vi "controllerVoltage.vi"(8 "error in (no error)":errorcluster) -> (0 "error out":errorcluster)   [LabVIEW 2018]
uses:
  Global_1259.vi
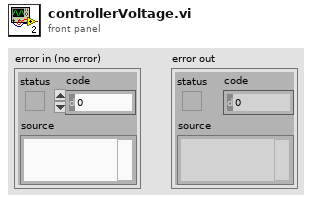
[diagram p1: front panel]
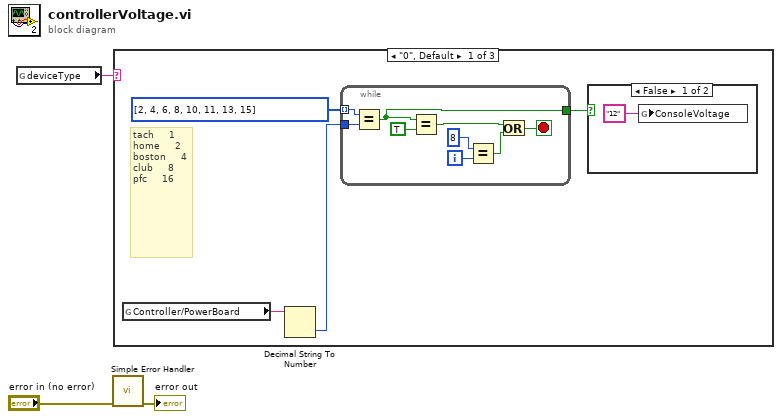
[diagram p0: block diagram]
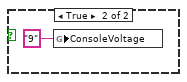
[diagram p2: hidden frame]
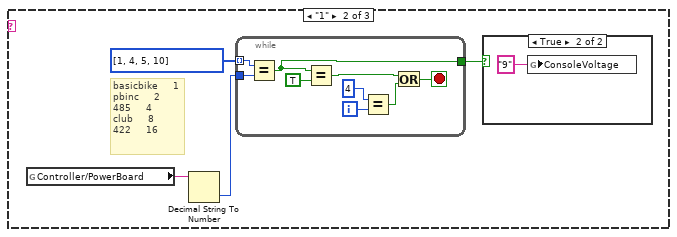
[diagram p3: hidden frame]
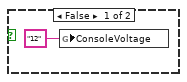
[diagram p4: hidden frame]
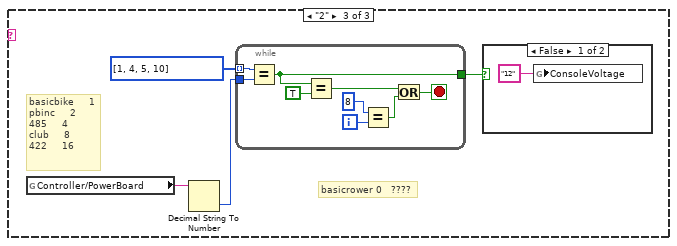
[diagram p5: hidden frame]
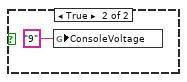
[diagram p6: hidden frame]
diagram:
  n1 = global read "Global_1259.vi" "deviceType"() -> (w3:string)
  n2 = call <vilib>:"Simple Error Handler.vi"("error in (no error)"="error in (no error)") -> ("error out"=→"error out":errorcluster)  [unwired: 4 in, 4 out]
  n3 = case shown="\"0\", Default" w3 {
    frame "0", Default {
      # "tach     1\nhome     2\nboston     4\nclub     8\npfc     16"
      n4 = global read "Global_1259.vi" "Controller/PowerBoard"() -> (w4:string)
      n5 = Decimal String To Number(string=w4) -> (number=w6:i32)  [unwired: 2 in, 1 out]
      n6 = while {
        tunnel: i32[] [2, 4, 6, 8, 10, 11, 13, 15] -> [w18] mode=indexing
        tunnel: w6 -> [w17]
        tunnel: [w10] -> w5
        i -> [w13]
        stop <- w11 stop-if-true
        n7 = Equal?(x=w18, y=w17) -> (x = y?=w10:bool)
        n8 = Equal?(x=w10, y=TRUE) -> (x = y?=w14:bool)
        n9 = Equal?(x=8, y=w13) -> (x = y?=w15:bool)
        n10 = Or(x=w14, y=w15) -> (x .or. y?=w11:bool)
      }
      n11 = case shown="False" w5 {
        frame False {
          n12 = global write "Global_1259.vi" "ConsoleVoltage"("12" ("ConsoleVoltage")) -> ()
        }
        frame True {
          n13 = global write "Global_1259.vi" "ConsoleVoltage"("9" ("ConsoleVoltage")) -> ()
        }
      }
    }
    frame "1" {
      # "basicbike     1\npbinc     2\n485     4\nclub     8\n422     16"
      n14 = global read "Global_1259.vi" "Controller/PowerBoard"() -> (w19:string)
      n15 = Decimal String To Number(string=w19) -> (number=w21:i32)  [unwired: 2 in, 1 out]
      n16 = while {
        tunnel: i32[] [1, 4, 5, 10] -> [w33] mode=indexing
        tunnel: w21 -> [w32]
        tunnel: [w25] -> w20
        i -> [w28]
        stop <- w26 stop-if-true
        n17 = Equal?(x=w33, y=w32) -> (x = y?=w25:bool)
        n18 = Equal?(x=w25, y=TRUE) -> (x = y?=w29:bool)
        n19 = Equal?(x=4, y=w28) -> (x = y?=w30:bool)
        n20 = Or(x=w29, y=w30) -> (x .or. y?=w26:bool)
      }
      n21 = case shown="True" w20 {
        frame False {
          n22 = global write "Global_1259.vi" "ConsoleVoltage"("12" ("ConsoleVoltage")) -> ()
        }
        frame True {
          n23 = global write "Global_1259.vi" "ConsoleVoltage"("9" ("ConsoleVoltage")) -> ()
        }
      }
    }
    frame "2" {
      # "basicrower 0   ????"
      # "basicbike     1\npbinc     2\n485     4\nclub     8\n422     16"
      n24 = global read "Global_1259.vi" "Controller/PowerBoard"() -> (w34:string)
      n25 = Decimal String To Number(string=w34) -> (number=w36:i32)  [unwired: 2 in, 1 out]
      n26 = while {
        tunnel: i32[] [1, 4, 5, 10] -> [w48] mode=indexing
        tunnel: w36 -> [w47]
        tunnel: [w40] -> w35
        i -> [w43]
        stop <- w41 stop-if-true
        n27 = Equal?(x=w48, y=w47) -> (x = y?=w40:bool)
        n28 = Equal?(x=w40, y=TRUE) -> (x = y?=w44:bool)
        n29 = Equal?(x=8, y=w43) -> (x = y?=w45:bool)
        n30 = Or(x=w44, y=w45) -> (x .or. y?=w41:bool)
      }
      n31 = case shown="False" w35 {
        frame False {
          n32 = global write "Global_1259.vi" "ConsoleVoltage"("12" ("ConsoleVoltage")) -> ()
        }
        frame True {
          n33 = global write "Global_1259.vi" "ConsoleVoltage"("9" ("ConsoleVoltage")) -> ()
        }
      }
    }
  }
